vi "Script_Extract_Wfms_Waits.vi"(7 "Script Text":string="script Pirenea2Excits1Acq4s\n   wait until scriptTrigger0 \n   wait 949940\n   generate AutLaserOn\n   wait 49000\n   generate AutLaserOnFilterOff\n   wait 1000\n   wait 600\n   generate AutLaserOnFilterOffTrapStart\n   wait 300\n   generate AutLaserOnFilterOffTrapStop\n   wait 2000\n   generate AutLaserOnFilterOn\n   wait 47100\n   generate AutLaserOff\n   wait 3950000\n   generate Excit\n   wait 1200\n   generate Excit\n   wait 1200\n   generate Acq\n   wait 1000000\n   generate FilterOff\n   wait 1000\n   generate FilterOffEmptyingStart\n   wait 1000000\n   generate FilterOffEmptyingStop\n   wait 2000\n   generate Zeros\nend script", 8 "error in (no error)":errorcluster, 10 "Script File":string="Pirenea2Excits1Acq4s.txt", 11 "Script Path":path=path "D:/PIRENEA/TECHNICAL/TIMING_SCRIPTS") -> (0 "error out":errorcluster, 1 "Table of All Wfms":string[](array[string]), 2 "Script Text Cleaned":string, 3 "Table of Loaded Wfms":string[](array[string]))   [LabVIEW 2018]
uses:
  Global_Variables.vi
  <vilib>/regexp/Match Regular Expression.xnode
panel:
  out "Table of Waits":string[](array[string])
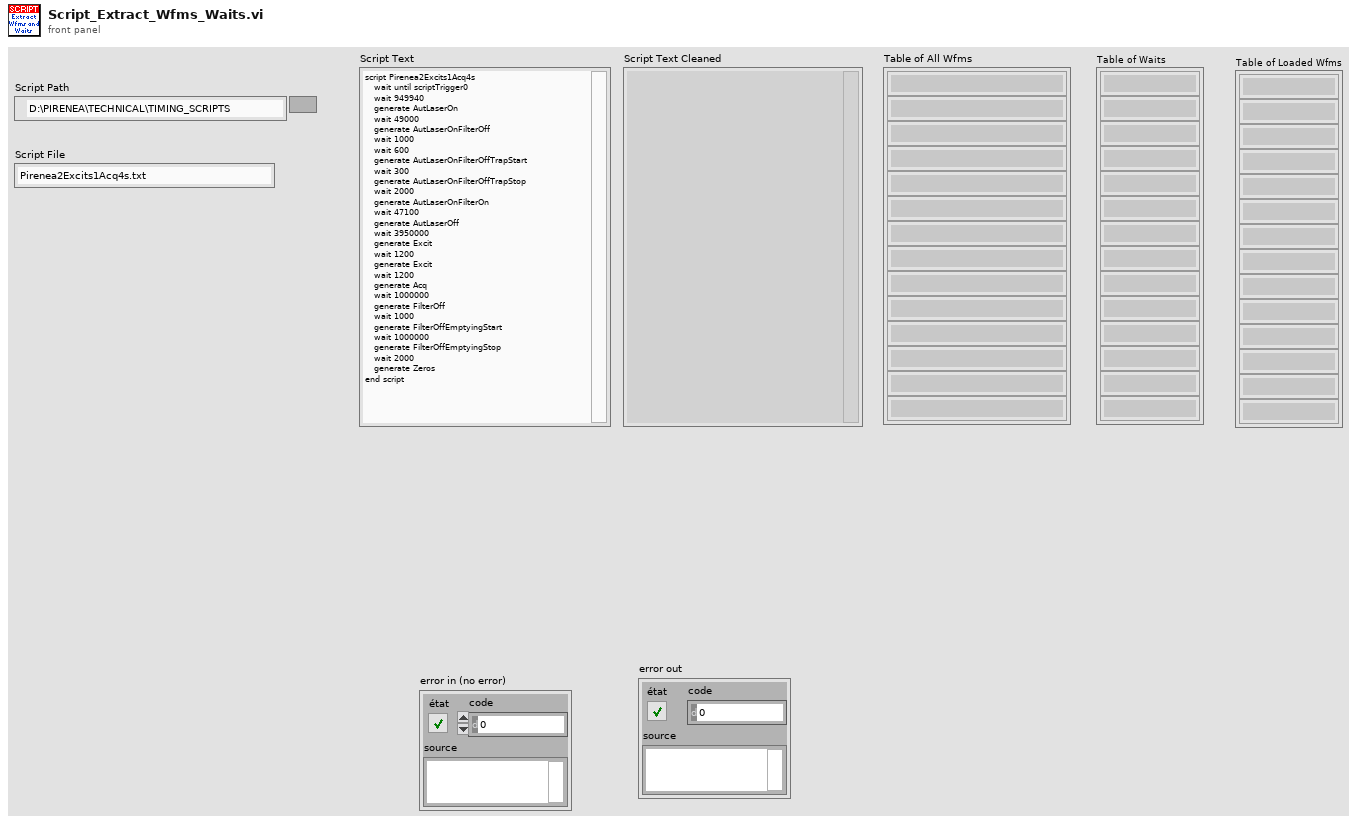
[diagram p1: front panel]
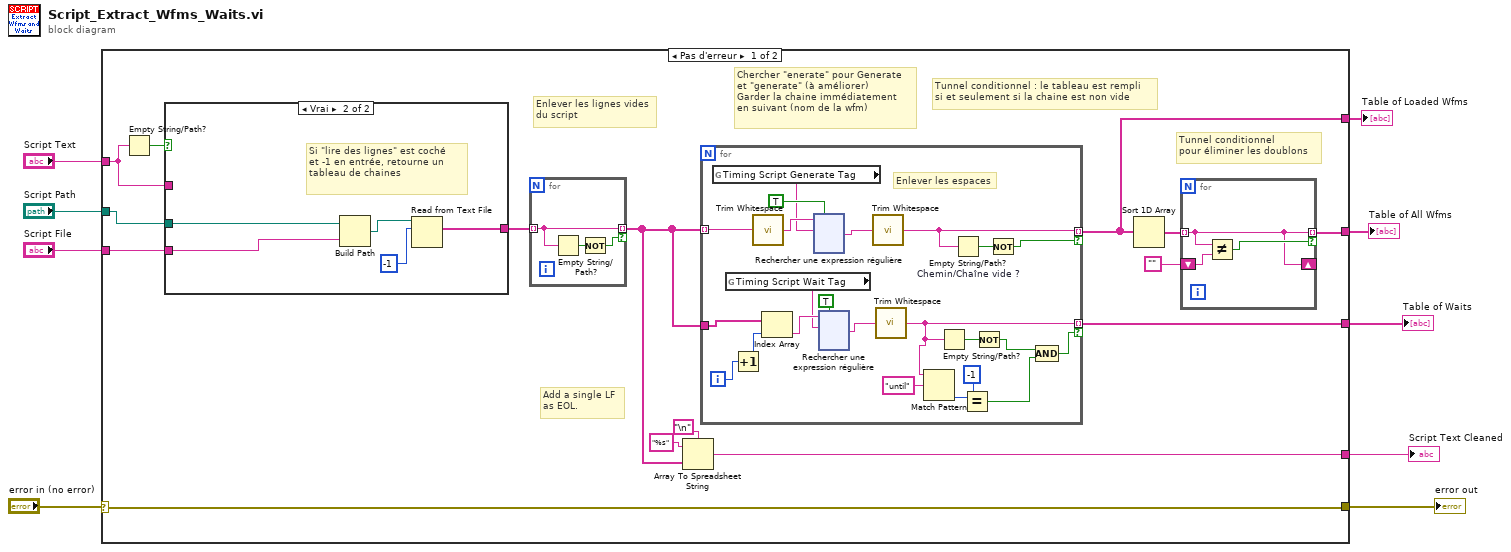
[diagram p0: block diagram]
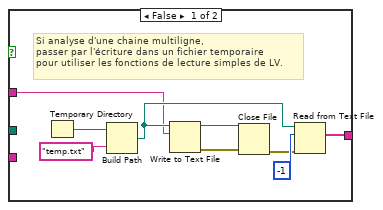
[diagram p2: hidden frame]
diagram:
  n1 = case shown="Pas d'erreur" "error in (no error)" {
    selector: "error in (no error)" -> [w17 w296]
    tunnel: [w24 _] -> w9
    tunnel: "Script Text" -> [w21 _]
    tunnel: [w12 _] -> w7
    tunnel: "Script Path" -> [w18 _]
    tunnel: "Script File" -> [w19 _]
    tunnel: [w17 w296] -> w4
    tunnel: [w15 _] -> w2
    tunnel: [w11 _] -> w1
    frame No Error {
      # "Add a single LF\nas EOL."
      # "Tunnel conditionnel\npour éliminer les doublons"
      # "Enlever les lignes vides\ndu script"
      # "Tunnel conditionnel : le tableau est rempli\nsi et seulement si la chaine est non vide"
      # "Chercher \"enerate\" pour Generate\net \"generate\" (à améliorer)\nGarder la chaine immédiatement\nen suivant (nom de la wfm)"
      n2 = Empty String/Path?(string/path=w21) -> (empty?=w20:bool)
      n3 = case shown="Vrai" w20 {
        tunnel: w19 -> [_ w44]
        tunnel: w18 -> [_ w43]
        tunnel: [w31 w40] -> w22
        tunnel: w21 -> [w32 _]
        frame False {
          # "Si analyse d'une chaine multiligne,\npasser par l'écriture dans un fichier temporaire\npour utiliser les fonctions de lecture simples de LV."
          n4 = Temporary Directory() -> (w38:path)
          n5 = Build Path(base path=w38, name or relative path="temp.txt" ("nom ou chemin relatif")) -> (appended path=w35:path)
          n6 = Write to Text File(file (use dialog)=w35, text=w32) -> (refnum out=w36:refnum<file>, error out=w37:errorcluster)  [unwired: 2 in, 1 out]
          n7 = Close File(refnum=w36, error in=w37) -> (error out=w33:errorcluster)  [unwired: 1 out]
          n8 = Read from Text File(file (use dialog)=w35, count=-1 ("nombre"), error in=w33) -> (text=w31:string[])  [unwired: 1 in, 3 out]
        }
        frame True {
          # "Si \"lire des lignes\" est coché\net -1 en entrée, retourne un tableau de chaines"
          n9 = Build Path(base path=w43, name or relative path=w44) -> (appended path=w42:path)
          n10 = Read from Text File(file (use dialog)=w42, count=-1 ("nombre")) -> (text=w40:string[])  [unwired: 2 in, 3 out]
        }
      }
      n11 = for {
        tunnel: w22 -> [w29] mode=indexing
        tunnel: [w29] -> w16 mode=indexing if=w28
        n12 = Empty String/Path?(string/path=w29) -> (empty?=w30:bool)
        n13 = Not(x=w30) -> (.not. x?=w28:bool)
      }
      n14 = Array To Spreadsheet String(delimiter (Tab)="\n", array=w16, 3:"%s" ("chaîne de format")) -> (spreadsheet string=w24:string)
      n15 = for {
        tunnel: w16 -> [w67] mode=indexing
        tunnel: [w63] -> w11 mode=indexing if=w64
        tunnel: w16 -> [w59]
        tunnel: [w51] -> w15 mode=indexing if=w45
        i -> [w58]
        # "Enlever les espaces"
        n16 = global read "Global_Variables.vi" "Timing Script Generate Tag"() -> (w60:string)
        n17 = global read "Global_Variables.vi" "Timing Script Wait Tag"() -> (w55:string)
        n18 = Increment(x=w58) -> (x+1=w57:i32)
        n19 = call <vilib>:"Trim Whitespace.vi"("string"=w67) -> ("trimmed string"=w62:string)  [unwired: 1 in]
        n20 = Index Array(array=w59, index=w57) -> (element=w56:string)
        n21 = xnode "Rechercher une expression régulière"("chaîne en entrée"=w62, "expression régulière"=w60, "ignorer la casse ? (F)"=TRUE) -> ("après la correspondance"=w66:string)  [unwired: 3 in, 4 out]
        n22 = xnode "Rechercher une expression régulière"("chaîne en entrée"=w56, "expression régulière"=w55, "ignorer la casse ? (F)"=TRUE) -> ("après la correspondance"=w52:string)  [unwired: 3 in, 4 out]
        n23 = call <vilib>:"Trim Whitespace.vi"("string"=w66) -> ("trimmed string"=w63:string)  [unwired: 1 in]
        n24 = call <vilib>:"Trim Whitespace.vi"("string"=w52) -> ("trimmed string"=w51:string)  [unwired: 1 in]
        n25 = Match Pattern(string=w51, regular expression="until" ("expression régulière")) -> (offset past match=w49:i32)  [unwired: 1 in, 3 out]
        n26 = Empty String/Path? ("Chemin/Chaîne vide ?")(string/path=w51) -> (empty?=w53:bool)
        n27 = Empty String/Path? "Chemin/Chaîne vide ?"(string/path=w63) -> (empty?=w65:bool)
        n28 = Equal?(x=w49, y=-1) -> (x = y?=w47:bool)
        n29 = Not(x=w53) -> (.not. x?=w46:bool)
        n30 = Not(x=w65) -> (.not. x?=w64:bool)
        n31 = Compound Arithmetic op=AND ("Opérateur arithmétique")(w46, w47) -> (w45:bool)
      }
      n32 = Sort 1D Array(array=w11) -> (sorted array=w14:string[])
      n33 = for {
        tunnel: w14 -> [w25] mode=indexing
        shift-right: [w25] -> _
        shift-left: "" -> [w27]
        tunnel: [w25] -> w12 mode=indexing if=w26
        n34 = Not Equal?(x=w25, y=w27) -> (x != y?=w26:bool)
      }
    }
    frame Error {
    }
  }
  "Script Text Cleaned" <- w9
  "Table of All Wfms" <- w7
  "error out" <- w4
  "Table of Waits" <- w2
  "Table of Loaded Wfms" <- w1
